vi "oscillscope test.vi"() -> ()   [LabVIEW 2010]
uses:
  <vilib>/Analysis/NI_AALBase.lvlib
panel:
  out "waveform out 2":cluster{"t(0)":ext, "delta t":ext, ext[]} {"t(0)" format="%.2e"; "?" format="%.4e"; "delta t" format="%.2e"}
  out "String 2":string
  in  "operation (entire wfm:0) 2":i32(ring) items=["Read entire waveform", "Read waveform segment defined by STARTING and ENDING points", "Read waveform segment defined by vertical cursor locations"]
  in  "source (ch1:0) 2":i32(ring) items=["Channel 1", "Channel 2", "Reference 1", "Reference 2", "Math"]
  in  "ending point 2":ext=500.0
  in  "starting point 2":ext=1.0
  out "String":string
  out "XY Graph":cluster{dbl[], dbl[]}[](graph)
  in  "Stop?":bool
  out "error out":errorcluster
  out "waveform out":cluster{"t(0)":ext, "delta t":ext, ext[]} {"t(0)" format="%.2e"; "?" format="%.4e"; "delta t" format="%.2e"}
  in  "operation (entire wfm:0)":i32(ring) items=["Read entire waveform", "Read waveform segment defined by STARTING and ENDING points", "Read waveform segment defined by vertical cursor locations"]
  in  "source (ch1:0)":i32(ring) items=["Channel 1", "Channel 2", "Reference 1", "Reference 2", "Math"]
  in  "ending point":ext=500.0
  in  "starting point":ext=1.0
  out "returned waveform":cluster{dbl, dbl, ext[]}(graph)
  in  "iteration (0:initialize)":i32
  in  "GPIB address":i16
  in  "error in (no error)":errorcluster
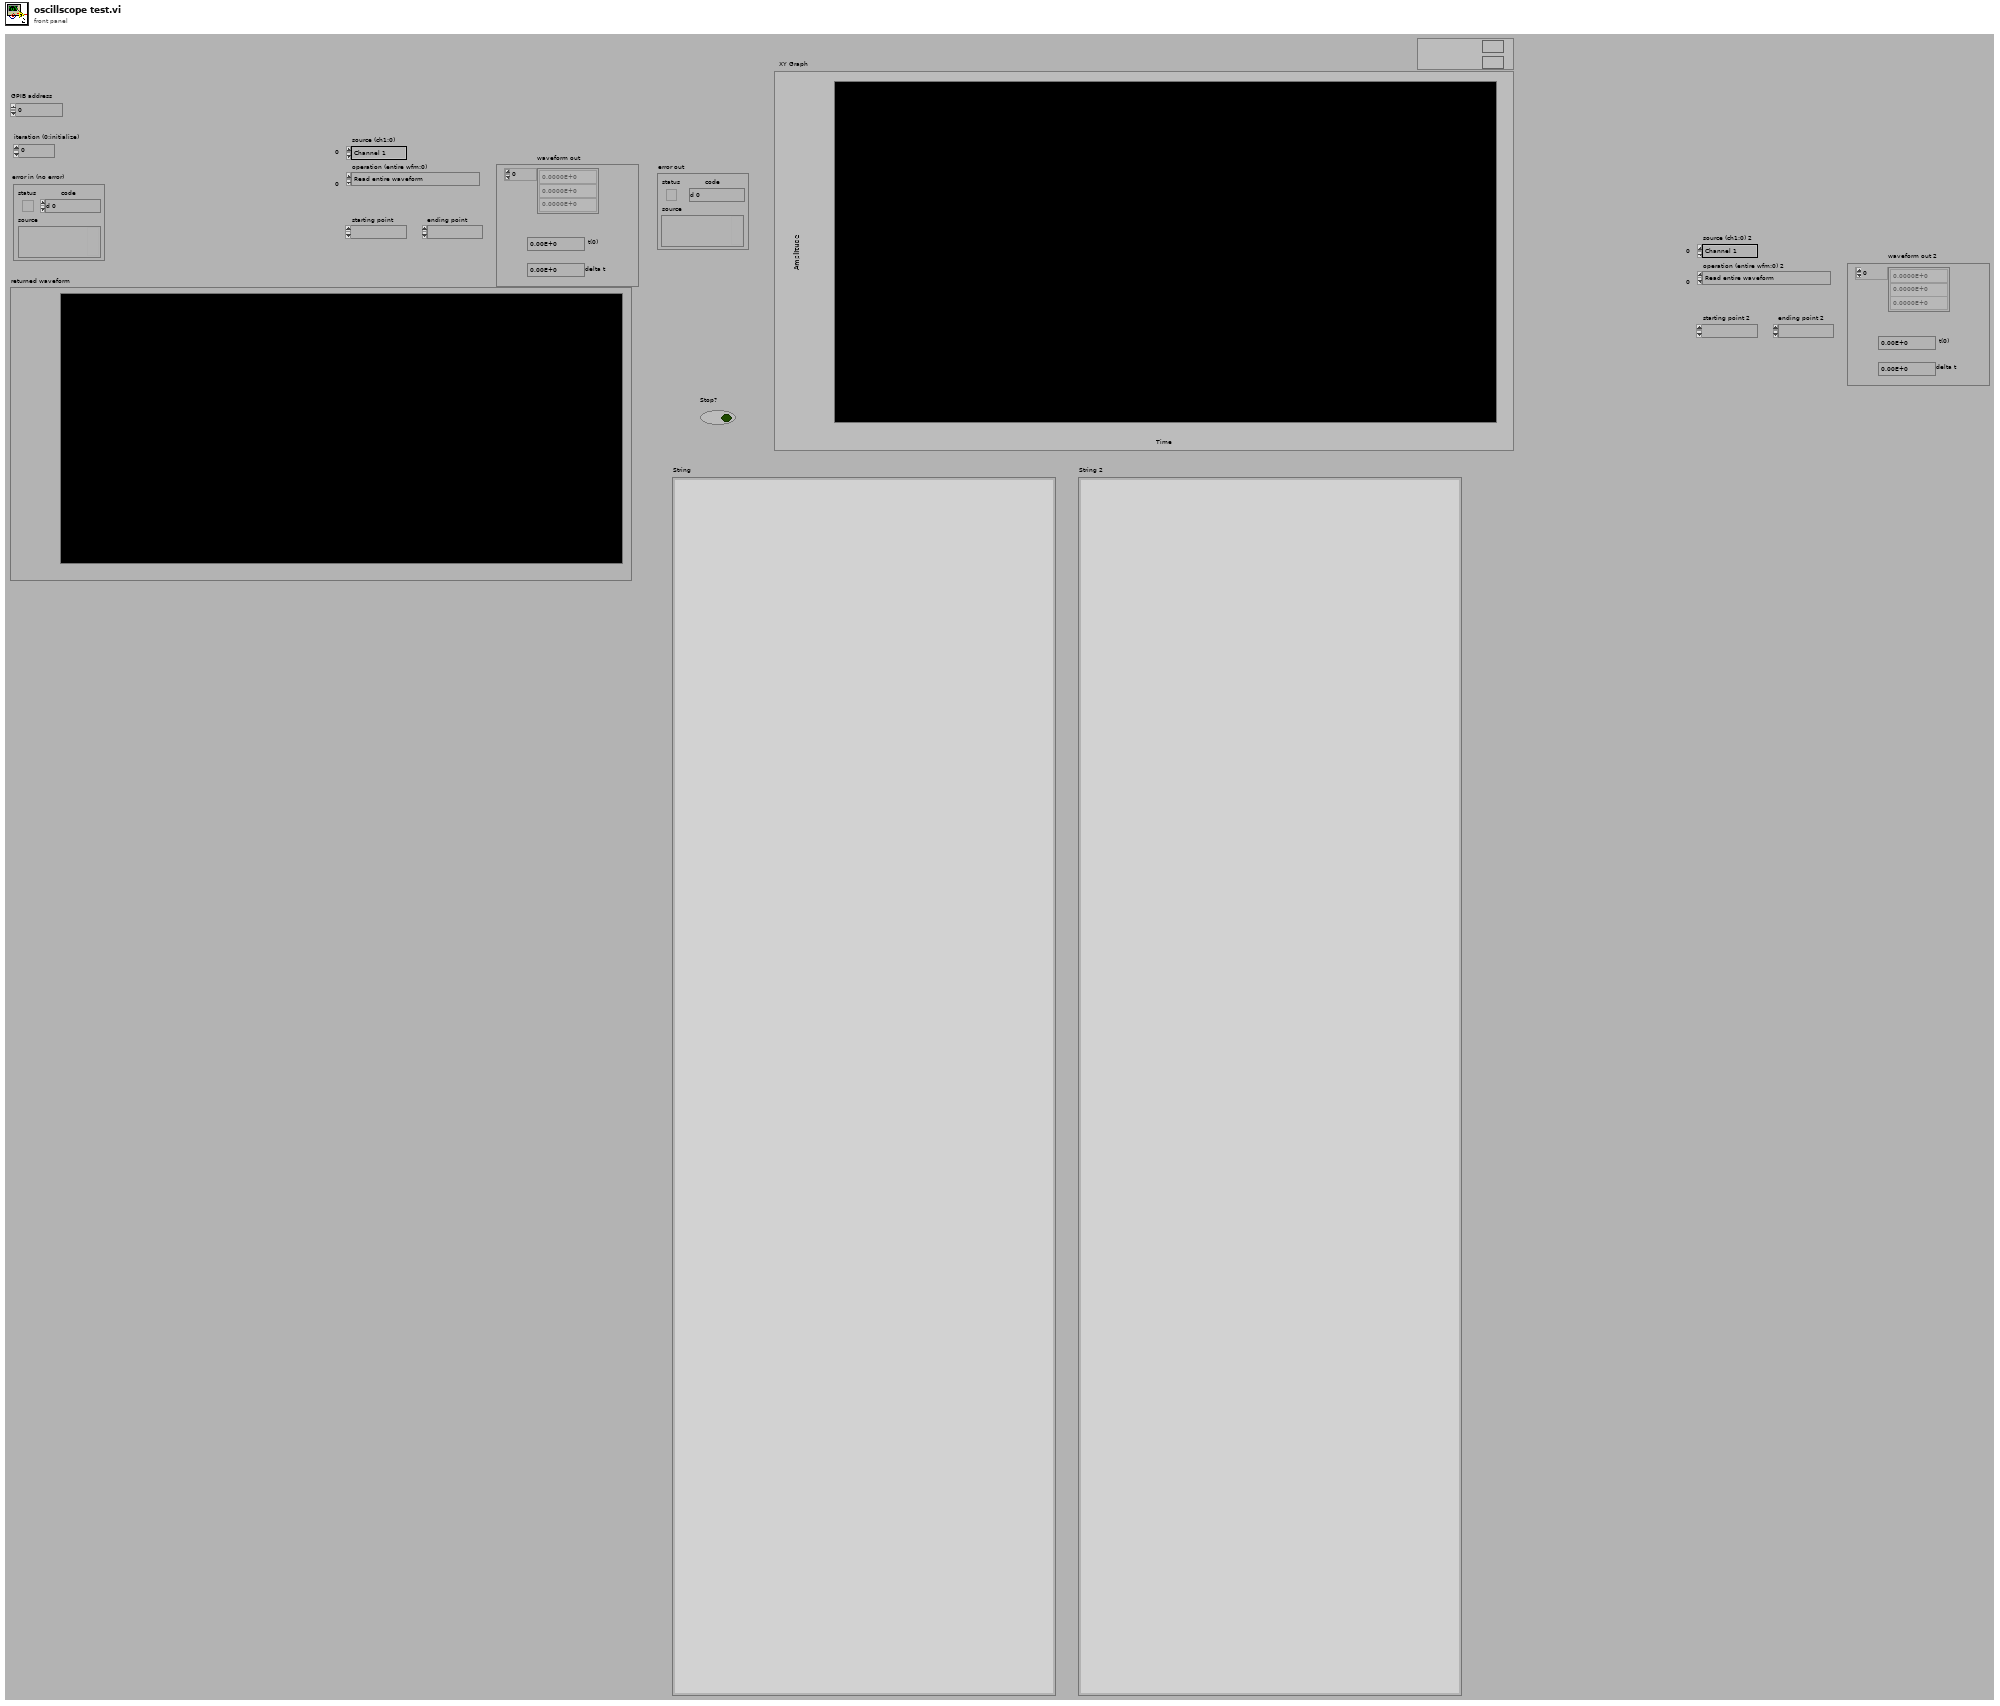
[diagram p1: front panel]
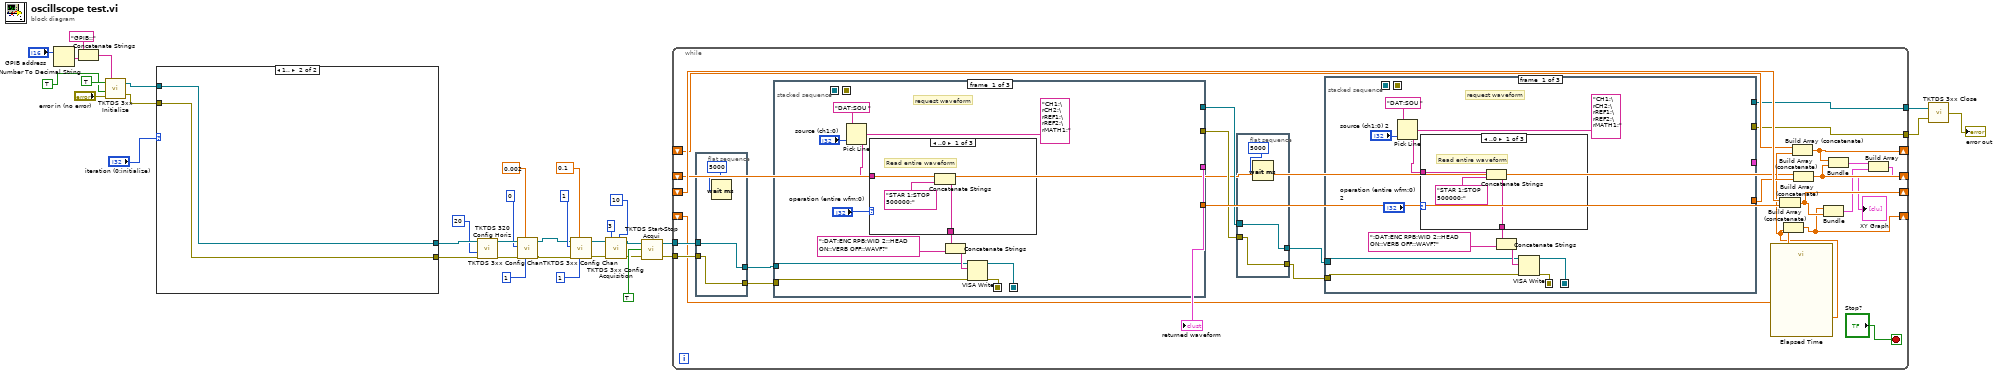
[diagram p0: block diagram]
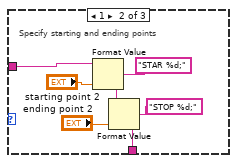
[diagram p2: hidden frame]
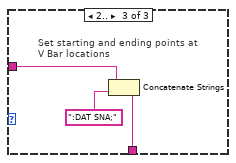
[diagram p3: hidden frame]
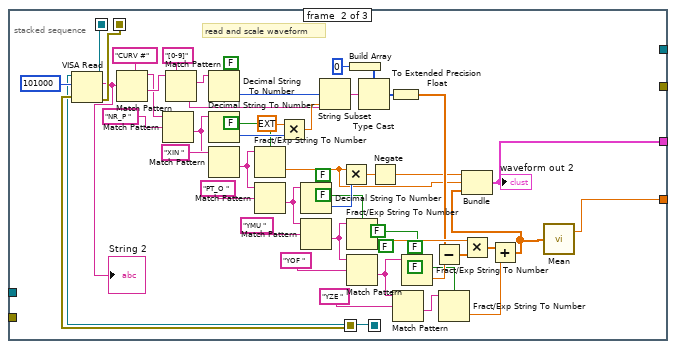
[diagram p4: hidden frame]
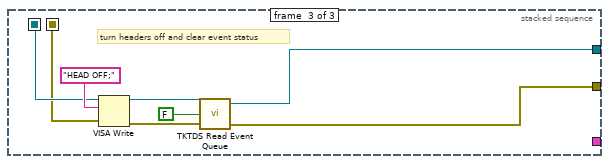
[diagram p5: hidden frame]
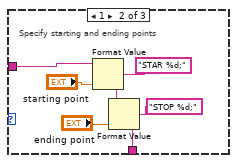
[diagram p6: hidden frame]
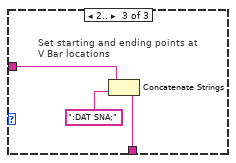
[diagram p7: hidden frame]
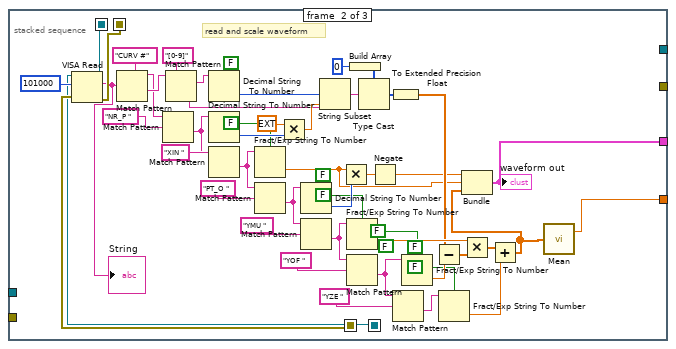
[diagram p8: hidden frame]
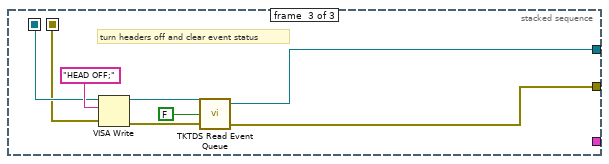
[diagram p9: hidden frame]
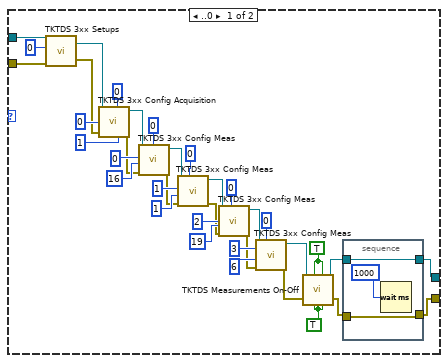
[diagram p10: hidden frame]
diagram:
  n1 = Number To Decimal String(number="GPIB address") -> (decimal integer string=w31:string)  [unwired: 1 in]
  n2 = Concatenate Strings("GPIB::", w31) -> (w32:string)
  n3 = call <instrlib>:"TKTDS 3xx Initialize.vi"("error in (no error)"="error in (no error)", "reset"=TRUE, "ID query"=TRUE, "instrument descripter (GPIB::1)"=w32) -> ("error out"=w26:errorcluster, "VISA session"=w27:refnum<visa-resource-name>)
  n4 = case shown="1.." "iteration (0:initialize)" {
    tunnel: w27 -> [w47 w76]
    tunnel: w26 -> [w46 w75]
    tunnel: [w38 w76] -> w24
    tunnel: [w36 w75] -> w23
    frame ..0 {
      w42 = TRUE
      w43 = TRUE
      n5 = call <instrlib>:"TKTDS 3xx Setups.vi"("error in (no error)"=w46, "operation (autosetup:0)"=0, "VISA session"=w47) -> ("error out"=w40:errorcluster, "dup VISA session"=w41:refnum<visa-resource-name>)  [unwired: 1 in]
      n6 = call <instrlib>:"TKTDS 3xx Config Acquisition.vi"("VISA session"=w41, "acqusition mode\n(sample:0)"=0, "error in (no error)"=w40, "# to average"=0, "number"=1) -> ("dup VISA session"=w68:refnum<visa-resource-name>, "error out"=w52:errorcluster)  [unwired: 4 in]
      n7 = call <instrlib>:"TKTDS 3xx Config Meas.vi"("source 1 (ch1:0)"=u8 0, "error in (no error)"=w52, "measurement type\n(period:0)"=16, "measurement to define\n(meas1:0)"=u8 0, "VISA session"=w68) -> ("error out"=w51:errorcluster, "dup VISA session"=w69:refnum<visa-resource-name>)  [unwired: 4 in]
      n8 = call <instrlib>:"TKTDS 3xx Config Meas.vi"("source 1 (ch1:0)"=0, "error in (no error)"=w51, "measurement type\n(period:0)"=1, "measurement to define\n(meas1:0)"=1, "VISA session"=w69) -> ("error out"=w50:errorcluster, "dup VISA session"=w70:refnum<visa-resource-name>)  [unwired: 4 in]
      n9 = call <instrlib>:"TKTDS 3xx Config Meas.vi"("source 1 (ch1:0)"=0, "error in (no error)"=w50, "measurement type\n(period:0)"=19, "measurement to define\n(meas1:0)"=2, "VISA session"=w70) -> ("error out"=w49:errorcluster, "dup VISA session"=w71:refnum<visa-resource-name>)  [unwired: 4 in]
      n10 = call <instrlib>:"TKTDS 3xx Config Meas.vi"("source 1 (ch1:0)"=0, "error in (no error)"=w49, "measurement type\n(period:0)"=6, "measurement to define\n(meas1:0)"=3, "VISA session"=w71) -> ("error out"=w44:errorcluster, "dup VISA session"=w48:refnum<visa-resource-name>)  [unwired: 4 in]
      n11 = call <instrlib>:"TKTDS Measurements On-Off.vi"("error in (no error)"=w44, "meas. 3"=w42, "meas. 4"=w42, "VISA session"=w48, "meas. 1"=w43, "meas. 2"=w43) -> ("error out"=w37:errorcluster, "dup VISA session"=w39:refnum<visa-resource-name>)
      n12 = stacked-sequence {
        tunnel: w39 -> [w73]
        tunnel: [w73] -> w38
        tunnel: [w72] -> w36
        tunnel: w37 -> [w72]
        frame #0 {
          n13 = Wait (ms)(milliseconds to wait=u32 1000) -> ()  [unwired: 1 out]
        }
      }
    }
    frame 1.. {
    }
  }
  n14 = call <instrlib>:"TKTDS 320 Config Horiz.vi"("error in (no error)"=w23, "main scaling\n(500us/div:15)"=20, "VISA session"=w24) -> ("error out"=w19:errorcluster, "dup VISA session"=w21:refnum<visa-resource-name>)  [unwired: 4 in]
  n15 = call <instrlib>:"TKTDS 3xx Config Chan.vi"("coupling\n(AC:0)"=1, "scaling"=0.002, "error in (no error)"=w19, "channel to set\n(ch1:0)"=0, "VISA session"=w21) -> ("error out"=w3:errorcluster, "dup VISA session"=w4:refnum<visa-resource-name>)  [unwired: 4 in, 1 out]
  n16 = call <instrlib>:"TKTDS 3xx Config Chan.vi"("coupling\n(AC:0)"=1, "scaling"=0.1, "error in (no error)"=w3, "channel to set\n(ch1:0)"=1, "VISA session"=w4) -> ("error out"=w2:errorcluster, "dup VISA session"=w1:refnum<visa-resource-name>)  [unwired: 4 in, 1 out]
  n17 = call <instrlib>:"TKTDS 3xx Config Acquisition.vi"("VISA session"=w1, "acqusition mode\n(sample:0)"=3, "error in (no error)"=w2, "# to average"=10) -> ("dup VISA session"=w16:refnum<visa-resource-name>, "error out"=w15:errorcluster)  [unwired: 5 in]
  n18 = call <instrlib>:"TKTDS Start-Stop Acqui.vi"("error in (no error)"=w15, "run/stop"=TRUE, "VISA session"=w16) -> ("error out"=w11:errorcluster, "dup VISA session"=w12:refnum<visa-resource-name>)  [unwired: 1 out]
  n19 = while {
    tunnel: w12 -> [w101]
    tunnel: w11 -> [w100]
    tunnel: [w83] -> w10
    tunnel: [w82] -> w9
    shift-right: [w93] -> _
    shift-left: _ -> [w95]
    shift-right: [w92] -> _
    shift-left: _ -> [w94]
    shift-right: [w81] -> _
    shift-left: _ -> [w85]
    shift-right: [w80] -> _
    shift-left: _ -> [w84]
    stop <- "Stop?" stop-if-true
    n20 = flat-sequence {
      tunnel: w101 -> [w189]
      tunnel: w100 -> [w190]
      tunnel: [w190] -> w99
      tunnel: [w189] -> w98
      frame #0 {
        n21 = Wait (ms)(milliseconds to wait=5000) -> ()  [unwired: 1 out]
      }
    }
    n22 = stacked-sequence {
      seq-local: [w195 _ _] -> [_ w228 _]
      seq-local: [w194 _ _] -> [_ w224 _]
      seq-local: [_ w227 _] -> [_ _ w271]
      seq-local: [_ w226 _] -> [_ _ w270]
      tunnel: w98 -> [w193 _ _]
      tunnel: w99 -> [w192 _ _]
      tunnel: [_ w219 _] -> w102
      tunnel: [_ _ w266] -> w90
      tunnel: [_ _ w265] -> w91
      tunnel: [_ w217 _] -> w96
      frame #0 {
        # "request waveform"
        n23 = Pick Line(string ("")="DAT:SOU ", multi-line string="CH1;\rCH2;\rREF1;\rREF2;\rMATH1;", line index="source (ch1:0)") -> (output string=w191:string)
        n24 = case shown="..0" "operation (entire wfm:0)" {
          tunnel: [w204 w208 w214] -> w198
          tunnel: w191 -> [w205 w209 w215]
          frame ..0 {
            # "Read entire waveform"
            n25 = Concatenate Strings(w205, "STAR 1;STOP 500000;") -> (w204:string)
          }
          frame 1 {
            # "Specify starting and ending points"
            n26 = Format Value(string ("")=w209, format string="STAR %d;", value (0)="starting point") -> (output string=w210:string)
            n27 = Format Value(string ("")=w210, format string="STOP %d;", value (0)="ending point") -> (output string=w208:string)
          }
          frame 2.. {
            # "Set starting and ending points at V Bar locations"
            n28 = Concatenate Strings(w215, ":DAT SNA;") -> (w214:string)
          }
        }
        n29 = Concatenate Strings(w198, ":DAT:ENC RPB;WID 2;:HEAD ON;:VERB OFF;:WAVF?") -> (w196:string)
        n30 = VISA Write(VISA resource name=w193, write buffer=w196, error in (no error)=w192) -> (VISA resource name out=w194:refnum<visa-resource-name>, error out=w195:errorcluster)  [unwired: 1 out]
      }
      frame #1 {
        (unwired) FALSE ("use system decimal point (T)")
        (unwired) FALSE ("use system decimal point (T)")
        (unwired) FALSE ("use system decimal point (T)")
        (unwired) FALSE ("use system decimal point (T)")
        # "read and scale waveform"
        n31 = VISA Read(VISA resource name=w224, byte count=101000, error in (no error)=w228) -> (VISA resource name out=w227:refnum<visa-resource-name>, read buffer=w216:string, error out=w226:errorcluster)  [unwired: 1 out]
        "String" <- w216
        n32 = Match Pattern(string=w216, regular expression="CURV #") -> (before substring=w236:string, after substring=w243:string)  [unwired: 1 in, 2 out]
        n33 = Match Pattern(string=w236, regular expression="NR_P ") -> (after substring=w237:string)  [unwired: 1 in, 3 out]
        n34 = Match Pattern(string=w243, regular expression="[0-9]") -> (match substring=w238:string, after substring=w239:string)  [unwired: 1 in, 2 out]
        n35 = Decimal String To Number(string=w238) -> (number=w240:i32)  [unwired: 2 in, 1 out]
        n36 = Decimal String To Number(string=w237) -> (number=w241:i32)  [unwired: 2 in, 1 out]
        n37 = Match Pattern(string=w237, regular expression="XIN ") -> (after substring=w249:string)  [unwired: 1 in, 3 out]
        n38 = Fract/Exp String To Number(use system decimal point (T)=FALSE, string=w249) -> (number=w229:dbl)  [unwired: 2 in, 1 out]
        n39 = Match Pattern(string=w249, regular expression="PT_O ") -> (after substring=w244:string)  [unwired: 1 in, 3 out]
        n40 = Multiply(x=ext 2.0, y=w241) -> (x*y=w242:ext)
        n41 = Decimal String To Number(string=w244) -> (number=w246:i32)  [unwired: 2 in, 1 out]
        n42 = Match Pattern(string=w244, regular expression="YMU ") -> (after substring=w252:string)  [unwired: 1 in, 3 out]
        n43 = String Subset(string=w239, offset (0)=w240, length (rest)=w242) -> (substring=w232:string)
        n44 = Multiply(x=w229, y=w246) -> (x*y=w262:dbl)
        n45 = Fract/Exp String To Number(use system decimal point (T)=FALSE, string=w252) -> (number=w259:dbl)  [unwired: 2 in, 1 out]
        n46 = Match Pattern(string=w252, regular expression="YOF ") -> (after substring=w255:string)  [unwired: 1 in, 3 out]
        n47 = Build Array(u16 0) -> (w234:u16[])
        n48 = Type Cast(type=w234, x=w232) -> (*(type *) &x=w235:u16[])
        n49 = Negate(x=w262) -> (-x=w230:dbl)
        n50 = To Extended Precision Float(1:w235) -> (0:w231:ext[])
        n51 = Match Pattern(string=w255, regular expression="YZE ") -> (after substring=w254:string)  [unwired: 1 in, 3 out]
        n52 = Fract/Exp String To Number(use system decimal point (T)=FALSE, string=w255) -> (number=w260:dbl)  [unwired: 2 in, 1 out]
        n53 = Subtract(x=w231, y=w260) -> (x-y=w258:ext[])
        n54 = Fract/Exp String To Number(use system decimal point (T)=FALSE, string=w254) -> (number=w261:dbl)  [unwired: 2 in, 1 out]
        n55 = Multiply(x=w259, y=w258) -> (x*y=w257:ext[])
        n56 = Add(x=w257, y=w261) -> (x+y=w218:ext[])
        n57 = Bundle(w230, w229, w218) -> (w219:cluster{dbl, dbl, ext[]})  [unwired: 1 in]
        "waveform out" <- w219
        n58 = call <vilib>:"Mean.vi"("X"=w218) -> ("mean"=w217:dbl)  [unwired: 1 out]
      }
      frame #2 {
        # "turn headers off and clear event status"
        n59 = VISA Write(VISA resource name=w271, write buffer="HEAD OFF;", error in (no error)=w270) -> (VISA resource name out=w267:refnum<visa-resource-name>, error out=w268:errorcluster)  [unwired: 1 out]
        n60 = call "TKTDS Read Event Queue.vi"("error in (no error)"=w268, "function"=FALSE, "VISA session"=w267) -> ("error out"=w265:errorcluster, "dup VISA session"=w266:refnum<visa-resource-name>)  [unwired: 1 out]
      }
    }
    "returned waveform" <- w102
    n61 = flat-sequence {
      tunnel: w90 -> [w186]
      tunnel: w91 -> [w187]
      tunnel: [w187] -> w88
      tunnel: [w186] -> w89
      frame #0 {
        n62 = Wait (ms)(milliseconds to wait=5000) -> ()  [unwired: 1 out]
      }
    }
    n63 = stacked-sequence {
      seq-local: [w107 _ _] -> [_ w140 _]
      seq-local: [w106 _ _] -> [_ w136 _]
      seq-local: [_ w139 _] -> [_ _ w183]
      seq-local: [_ w138 _] -> [_ _ w182]
      tunnel: w89 -> [w105 _ _]
      tunnel: w88 -> [w104 _ _]
      tunnel: [_ w131 _] -> _
      tunnel: [_ _ w178] -> w83
      tunnel: [_ _ w177] -> w82
      tunnel: [_ w129 _] -> w87
      frame #0 {
        # "request waveform"
        n64 = Pick Line(string ("")="DAT:SOU ", multi-line string="CH1;\rCH2;\rREF1;\rREF2;\rMATH1;", line index="source (ch1:0) 2") -> (output string=w103:string)
        n65 = case shown="..0" "operation (entire wfm:0) 2" {
          tunnel: [w116 w120 w126] -> w110
          tunnel: w103 -> [w117 w121 w127]
          frame ..0 {
            # "Read entire waveform"
            n66 = Concatenate Strings(w117, "STAR 1;STOP 500000;") -> (w116:string)
          }
          frame 1 {
            # "Specify starting and ending points"
            n67 = Format Value(string ("")=w121, format string="STAR %d;", value (0)="starting point 2") -> (output string=w122:string)
            n68 = Format Value(string ("")=w122, format string="STOP %d;", value (0)="ending point 2") -> (output string=w120:string)
          }
          frame 2.. {
            # "Set starting and ending points at V Bar locations"
            n69 = Concatenate Strings(w127, ":DAT SNA;") -> (w126:string)
          }
        }
        n70 = Concatenate Strings(w110, ":DAT:ENC RPB;WID 2;:HEAD ON;:VERB OFF;:WAVF?") -> (w108:string)
        n71 = VISA Write(VISA resource name=w105, write buffer=w108, error in (no error)=w104) -> (VISA resource name out=w106:refnum<visa-resource-name>, error out=w107:errorcluster)  [unwired: 1 out]
      }
      frame #1 {
        (unwired) FALSE ("use system decimal point (T)")
        (unwired) FALSE ("use system decimal point (T)")
        (unwired) FALSE ("use system decimal point (T)")
        (unwired) FALSE ("use system decimal point (T)")
        # "read and scale waveform"
        n72 = VISA Read(VISA resource name=w136, byte count=101000, error in (no error)=w140) -> (VISA resource name out=w139:refnum<visa-resource-name>, read buffer=w128:string, error out=w138:errorcluster)  [unwired: 1 out]
        "String 2" <- w128
        n73 = Match Pattern(string=w128, regular expression="CURV #") -> (before substring=w148:string, after substring=w155:string)  [unwired: 1 in, 2 out]
        n74 = Match Pattern(string=w148, regular expression="NR_P ") -> (after substring=w149:string)  [unwired: 1 in, 3 out]
        n75 = Match Pattern(string=w155, regular expression="[0-9]") -> (match substring=w150:string, after substring=w151:string)  [unwired: 1 in, 2 out]
        n76 = Decimal String To Number(string=w150) -> (number=w152:i32)  [unwired: 2 in, 1 out]
        n77 = Decimal String To Number(string=w149) -> (number=w153:i32)  [unwired: 2 in, 1 out]
        n78 = Match Pattern(string=w149, regular expression="XIN ") -> (after substring=w161:string)  [unwired: 1 in, 3 out]
        n79 = Fract/Exp String To Number(use system decimal point (T)=FALSE, string=w161) -> (number=w141:dbl)  [unwired: 2 in, 1 out]
        n80 = Match Pattern(string=w161, regular expression="PT_O ") -> (after substring=w156:string)  [unwired: 1 in, 3 out]
        n81 = Multiply(x=ext 2.0, y=w153) -> (x*y=w154:ext)
        n82 = Decimal String To Number(string=w156) -> (number=w158:i32)  [unwired: 2 in, 1 out]
        n83 = Match Pattern(string=w156, regular expression="YMU ") -> (after substring=w164:string)  [unwired: 1 in, 3 out]
        n84 = String Subset(string=w151, offset (0)=w152, length (rest)=w154) -> (substring=w144:string)
        n85 = Multiply(x=w141, y=w158) -> (x*y=w174:dbl)
        n86 = Fract/Exp String To Number(use system decimal point (T)=FALSE, string=w164) -> (number=w171:dbl)  [unwired: 2 in, 1 out]
        n87 = Match Pattern(string=w164, regular expression="YOF ") -> (after substring=w167:string)  [unwired: 1 in, 3 out]
        n88 = Build Array(u16 0) -> (w146:u16[])
        n89 = Type Cast(type=w146, x=w144) -> (*(type *) &x=w147:u16[])
        n90 = Negate(x=w174) -> (-x=w142:dbl)
        n91 = To Extended Precision Float(1:w147) -> (0:w143:ext[])
        n92 = Match Pattern(string=w167, regular expression="YZE ") -> (after substring=w166:string)  [unwired: 1 in, 3 out]
        n93 = Fract/Exp String To Number(use system decimal point (T)=FALSE, string=w167) -> (number=w172:dbl)  [unwired: 2 in, 1 out]
        n94 = Subtract(x=w143, y=w172) -> (x-y=w170:ext[])
        n95 = Fract/Exp String To Number(use system decimal point (T)=FALSE, string=w166) -> (number=w173:dbl)  [unwired: 2 in, 1 out]
        n96 = Multiply(x=w171, y=w170) -> (x*y=w169:ext[])
        n97 = Add(x=w169, y=w173) -> (x+y=w130:ext[])
        n98 = Bundle(w142, w141, w130) -> (w131:cluster{dbl, dbl, ext[]})  [unwired: 1 in]
        "waveform out 2" <- w131
        n99 = call <vilib>:"Mean.vi"("X"=w130) -> ("mean"=w129:dbl)  [unwired: 1 out]
      }
      frame #2 {
        # "turn headers off and clear event status"
        n100 = VISA Write(VISA resource name=w183, write buffer="HEAD OFF;", error in (no error)=w182) -> (VISA resource name out=w179:refnum<visa-resource-name>, error out=w180:errorcluster)  [unwired: 1 out]
        n101 = call "TKTDS Read Event Queue.vi"("error in (no error)"=w180, "function"=FALSE, "VISA session"=w179) -> ("error out"=w177:errorcluster, "dup VISA session"=w178:refnum<visa-resource-name>)  [unwired: 1 out]
      }
    }
    n102 = call "Elapsed Time"() -> ("Elapsed Time (s)"=w86:dbl)  [unwired: 12 in, 7 out]
    n103 = Build Array (concatenate)(w95, w96) -> (w93:dbl[])
    n104 = Build Array (concatenate)(w94, w86) -> (w92:dbl[])
    n105 = Build Array (concatenate)(w85, w86) -> (w81:dbl[])
    n106 = Build Array (concatenate)(w84, w87) -> (w80:dbl[])
    n107 = Bundle(w92, w93) -> (w78:cluster{dbl[], dbl[]})  [unwired: 1 in]
    n108 = Bundle(w81, w80) -> (w79:cluster{dbl[], dbl[]})  [unwired: 1 in]
    n109 = Build Array(w79, w78) -> (→"XY Graph":cluster{dbl[], dbl[]}[])
  }
  n110 = call <instrlib>:"TKTDS 3xx Close.vi"("error in (no error)"=w9, "VISA session"=w10) -> ("error out"=→"error out":errorcluster)
